vi "Insert element in QUEUE.vi"(8 "error in (no error)":errorcluster, 10 "Element":T1, 11 "Queue name":string) -> (0 "error out":errorcluster, 1 "timed out?":bool)   [LabVIEW 2023, in "Queues.lvlib"]
uses:
  Queues.lvlib
  DUTinfo.ctl
  DUTResult.ctl
  Queue Priority.ctl
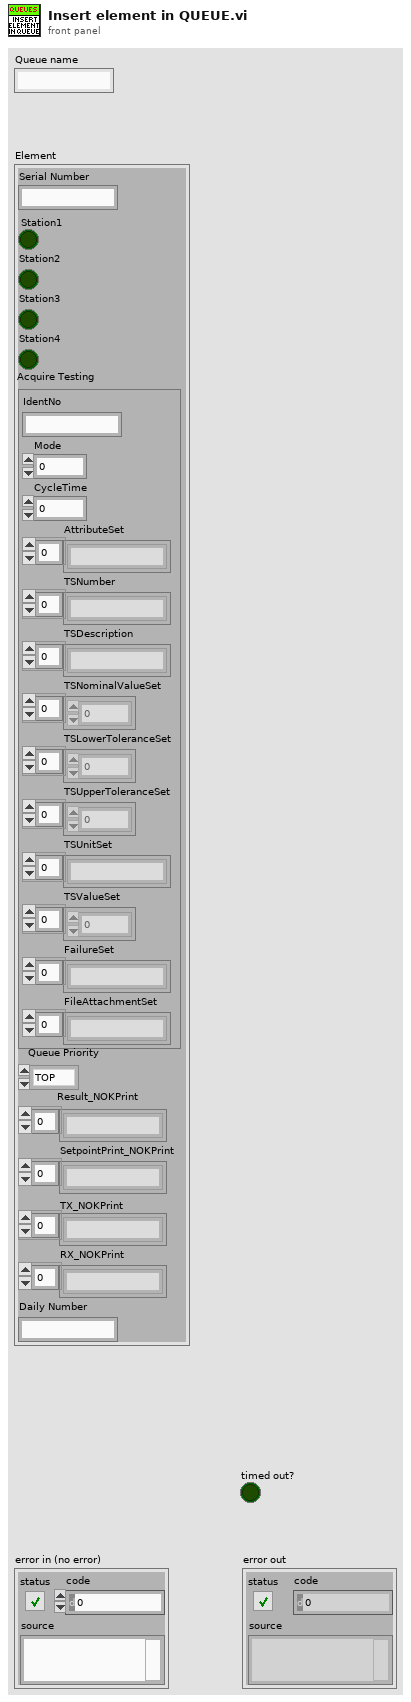
[diagram p1: front panel]
types:
  T1 = typedef "Queues.lvlib/DUTinfo.ctl" = cluster{"Serial Number":string, "Station1":bool, "Station2":bool, "Station3":bool, "Station4":bool, "Acquire Testing":T2, "Queue Priority":T3, "Result_NOKPrint":string[], "SetpointPrint_NOKPrint":string[], "TX_NOKPrint":string[], "RX_NOKPrint":string[], "Daily Number":string}
  T2 = typedef "Queues.lvlib/DUTResult.ctl" = cluster{"IdentNo":string, "Mode":dbl, "CycleTime":dbl, "AttributeSet":string[], "TSNumber":string[], "TSDescription":string[], "TSNominalValueSet":dbl[], "TSLowerToleranceSet":dbl[], "TSUpperToleranceSet":dbl[], "TSUnitSet":string[], "TSValueSet":dbl[], "FailureSet":string[], "FileAttachmentSet":string[]}
  T3 = typedef "Queues.lvlib/Queue Priority.ctl" = enum16{"TOP", "BOTTOM"}
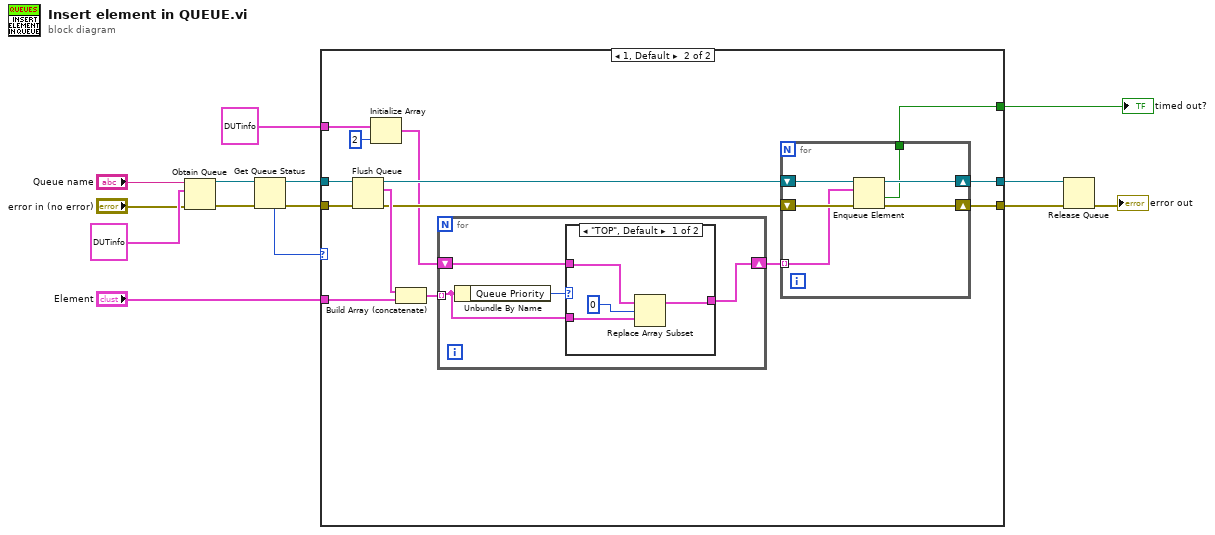
[diagram p0: block diagram]
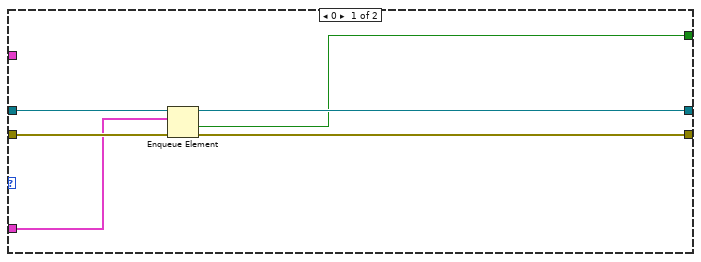
[diagram p2: hidden frame]
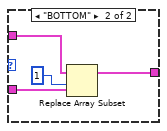
[diagram p3: hidden frame]
diagram:
  n1 = Obtain Queue(name (unnamed)="Queue name", element data type=T1 {"Serial Number"="", "Station1"=FALSE, "Station2"=FALSE, "Station3"=FALSE, "Station4"=FALSE, "Acquire Testing"={"IdentNo"="", "Mode"=0.0, "CycleTime"=0.0, "AttributeSet"=[], "TSNumber"=[], "TSDescription"=[], "TSNominalValueSet"=[], "TSLowerToleranceSet"=[], "TSUpperToleranceSet"=[], "TSUnitSet"=[], "TSValueSet"=[], "FailureSet"=[], "FileAttachmentSet"=[]}, "Queue Priority"=enum."TOP", "Result_NOKPrint"=[], "SetpointPrint_NOKPrint"=[], "TX_NOKPrint"=[], "RX_NOKPrint"=[], "Daily Number"=""} ("Element"), error in (no error)="error in (no error)") -> (queue out=w11:refnum<queue>, error out=w10:errorcluster)  [unwired: 2 in, 1 out]
  n2 = Get Queue Status(queue=w11, error in (no error)=w10) -> (queue out=w9:refnum<queue>, error out=w8:errorcluster, # elements in queue=w7:i32)  [unwired: 1 in, 5 out]
  n3 = case shown="1, Default" w7 {
    tunnel: w9 -> [w17 w34]
    tunnel: w8 -> [w16 w33]
    tunnel: [w20 w26] -> w6
    tunnel: [w19 w24] -> w5
    tunnel: [w18 w25] -> w4
    tunnel: "Element" -> [w15 w31]
    tunnel: T1 {"Serial Number"="", "Station1"=FALSE, "Station2"=FALSE, "Station3"=FALSE, "Station4"=FALSE, "Acquire Testing"={"IdentNo"="", "Mode"=0.0, "CycleTime"=0.0, "AttributeSet"=[], "TSNumber"=[], "TSDescription"=[], "TSNominalValueSet"=[], "TSLowerToleranceSet"=[], "TSUpperToleranceSet"=[], "TSUnitSet"=[], "TSValueSet"=[], "FailureSet"=[], "FileAttachmentSet"=[]}, "Queue Priority"=enum."TOP", "Result_NOKPrint"=[], "SetpointPrint_NOKPrint"=[], "TX_NOKPrint"=[], "RX_NOKPrint"=[], "Daily Number"=""} ("Element") -> [_ w23]
    frame 0 {
      n4 = Enqueue Element(queue=w17, element=w15, error in (no error)=w16) -> (queue out=w20:refnum<queue>, timed out?=w19:bool, error out=w18:errorcluster)  [unwired: 1 in]
    }
    frame 1, Default {
      n5 = Flush Queue(queue=w34, error in (no error)=w33) -> (queue out=w29:refnum<queue>, remaining elements=w32:T1[], error out=w28:errorcluster)
      n6 = Initialize Array(w23, 2 ("dimension size")) -> (w21:T1[])
      n7 = Build Array (concatenate)(w32, w31) -> (w30:T1[])
      n8 = for {
        tunnel: w30 -> [w43] mode=indexing
        shift-right: [w42] -> w27
        shift-left: w21 -> [w41]
        n9 = Unbundle By Name(w43) -> ("Queue Priority"=w44:T3)
        n10 = case shown="\"TOP\", Default" w44 {
          tunnel: w43 -> [w46 w52]
          tunnel: [w45 w51] -> w42
          tunnel: w41 -> [w47 w49]
          frame "TOP", Default {
            n11 = Replace Array Subset(array=w47, new element=w46, index=0) -> (w45:T1[])
          }
          frame "BOTTOM" {
            n12 = Replace Array Subset(array=w49, new element=w52, index=1) -> (w51:T1[])
          }
        }
      }
      n13 = for {
        tunnel: w27 -> [w38] mode=indexing
        shift-right: [w37] -> w26
        shift-left: w29 -> [w40]
        shift-right: [w36] -> w25
        shift-left: w28 -> [w39]
        tunnel: [w35] -> w24
        n14 = Enqueue Element(queue=w40, element=w38, error in (no error)=w39) -> (queue out=w37:refnum<queue>, timed out?=w35:bool, error out=w36:errorcluster)  [unwired: 1 in]
      }
    }
  }
  "timed out?" <- w5
  n15 = Release Queue(queue=w6, error in (no error)=w4) -> (error out=→"error out":errorcluster)  [unwired: 1 in, 2 out]
